vi "InsertPLCvalues.vi"(9 "172.18.214.225":string[](array[string]), 10 "172.18.214.231":string[](array[string]), 11 "Array":T1(array[cluster])) -> (2 "OutputValues":T1(array[cluster]))   [LabVIEW 2014]
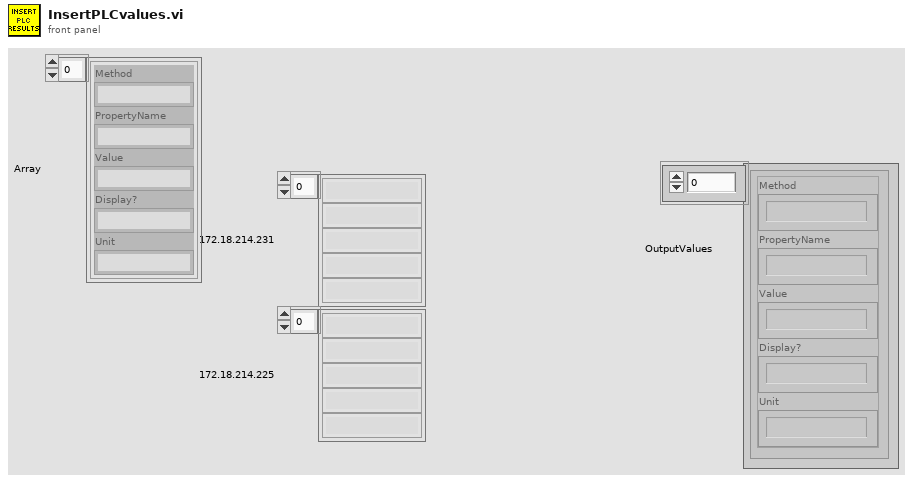
[diagram p1: front panel]
types:
  T1 = cluster{"Method":string, "PropertyName":string, "Value":string, "Display?":string, "Unit":string}[]
  T2 = cluster{"Method":string, "PropertyName":string, "Value":string, "Display?":string, "Unit":string}
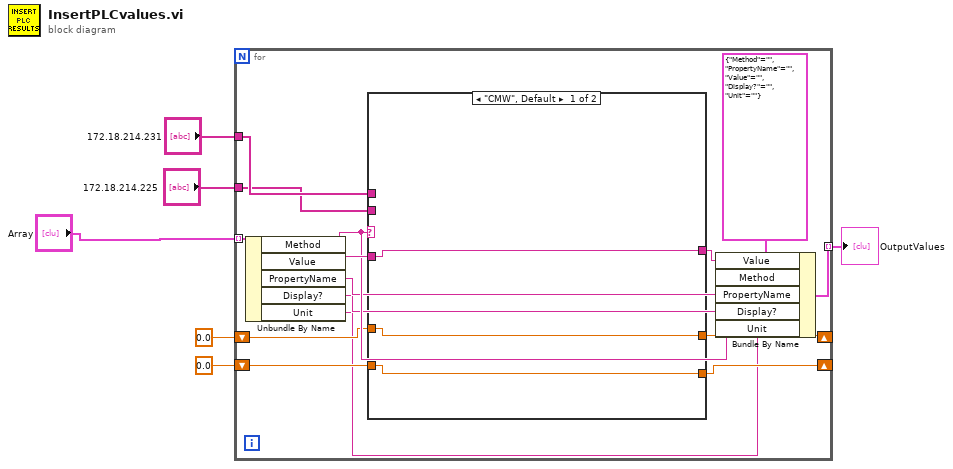
[diagram p0: block diagram]
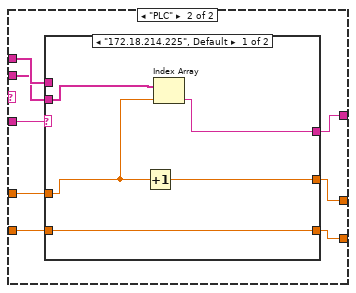
[diagram p2: hidden frame]
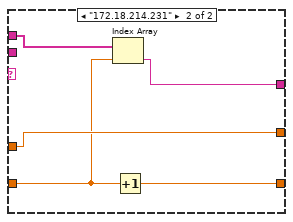
[diagram p3: hidden frame]
diagram:
  n1 = for {
    tunnel: "Array" -> [w21] mode=indexing
    tunnel: [w19] -> w2 mode=indexing
    tunnel: "172.18.214.231" -> [w14]
    tunnel: "172.18.214.225" -> [w13]
    shift-right: [w10] -> _
    shift-left: 0.0 -> [w11]
    shift-right: [w8] -> _
    shift-left: 0.0 -> [w9]
    n2 = Unbundle By Name(w21) -> ("Method"=w17:string, "Value"=w18:string, "PropertyName"=w16:string, "Display?"=w15:string, "Unit"=w7:string)
    n3 = case shown="\"CMW\", Default" w17 {
      tunnel: w18 -> [w24 w32]
      tunnel: [w24 w29] -> w12
      tunnel: w14 -> [_ w31]
      tunnel: w13 -> [_ w30]
      tunnel: w11 -> [w23 w28]
      tunnel: [w23 w27] -> w10
      tunnel: w9 -> [w22 w26]
      tunnel: [w22 w25] -> w8
      frame "CMW", Default {
      }
      frame "PLC" {
        n4 = case shown="\"172.18.214.225\", Default" w32 {
          tunnel: w31 -> [_ w41]
          tunnel: w30 -> [w36 _]
          tunnel: [w37 w42] -> w29
          tunnel: w28 -> [w34 w39]
          tunnel: [w35 w39] -> w27
          tunnel: w26 -> [w33 w38]
          tunnel: [w33 w40] -> w25
          frame "172.18.214.225", Default {
            n5 = Increment(x=w34) -> (x+1=w35:dbl)
            n6 = Index Array(array=w36, index=w34) -> (element=w37:string)
          }
          frame "172.18.214.231" {
            n7 = Index Array(array=w41, index=w38) -> (element=w42:string)
            n8 = Increment(x=w38) -> (x+1=w40:dbl)
          }
        }
      }
    }
    n9 = Bundle By Name(cluster=T2 {"Method"="", "PropertyName"="", "Value"="", "Display?"="", "Unit"=""} ("input cluster"), "Value"=w12, "Method"=w17, "PropertyName"=w16, "Display?"=w15, "Unit"=w7) -> (w19:T2)
  }
  "OutputValues" <- w2
